vi "Read ProjectItem Refnum.vi"(11 "ProjectItem in":refnum<class "ProjectItem.lvclass">) -> (2 "ProjectItem Refnum":refnum<vi>, 3 "ProjectItem out":refnum<class "ProjectItem.lvclass">)   [LabVIEW 2016, in "ProjectItem.lvclass"]
uses:
  ProjectItem.lvclass
  ProjectItem.lvclass/ProjectItem.ctl
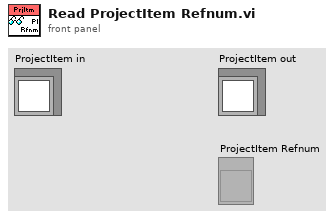
[diagram p1: front panel]
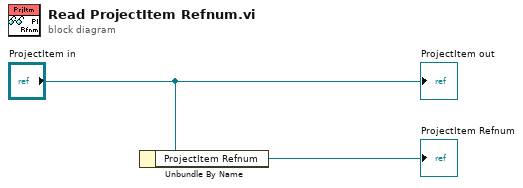
[diagram p0: block diagram]
diagram:
  n1 = Unbundle By Name("ProjectItem in") -> ("ProjectItem Refnum"=→"ProjectItem Refnum":refnum<vi>)
  "ProjectItem out" <- "ProjectItem in"
